vi "Config Trig Pos and Delay.vi"(0 "VISA resource name":refnum<visa-resource-name>, 5 "Trigger Position (0)":u16 max=100 step=1, 7 "Trigger Delay (0us)":dbl min=0.0 max=1000000.0 step=0.1 format="%.1f", 11 "error in (no error)":errorcluster) -> (4 "VISA resource name out":refnum<visa-resource-name>, 15 "error out":errorcluster)   [LabVIEW 2013, in "Yokogawa.lvlib" / "Yokogawa PZ4000.lvlib"]
doc: "This VI sends the Trigger command to the PZ4000.\nConfiguration Functions are Trigger Position, and Trigger Delay."
uses:
  Yokogawa PZ4000.lvlib
panel:
  # "us"
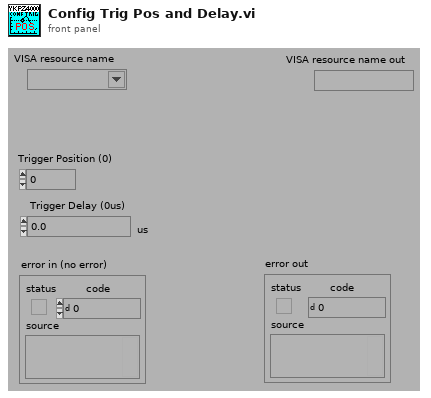
[diagram p1: front panel]
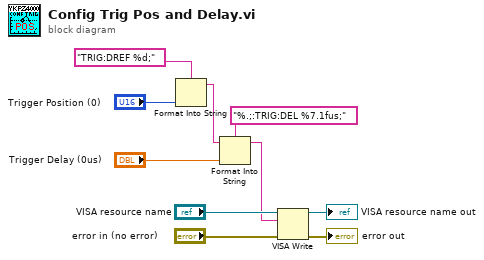
[diagram p0: block diagram]
diagram:
  n1 = Format Into String(format string="TRIG:DREF %d;", "Trigger Position (0)") -> (resulting string=w2:string)  [unwired: 2 in, 1 out]
  n2 = Format Into String(format string="%.;:TRIG:DEL %7.1fus;", initial string=w2, "Trigger Delay (0us)") -> (resulting string=w1:string)  [unwired: 1 in, 1 out]
  n3 = VISA Write(VISA resource name="VISA resource name", write buffer=w1, error in (no error)="error in (no error)") -> (VISA resource name out=→"VISA resource name out":refnum<visa-resource-name>, error out=→"error out":errorcluster)  [unwired: 1 out]
